vi "generate_longer_time_data.vi"(6 "new element":dbl[][](array[numeric]), 8 "Number of Samples":i32=100, 9 "横轴（显示时长）":dbl=1000.0, 10 "Sample Rate":dbl=1000.0, 11 "old array":dbl[][](array[numeric])) -> (0 "new array":dbl[][](array[numeric]), 3 "data":waveform(dbl)[](array[waveform]))   [LabVIEW 2024]
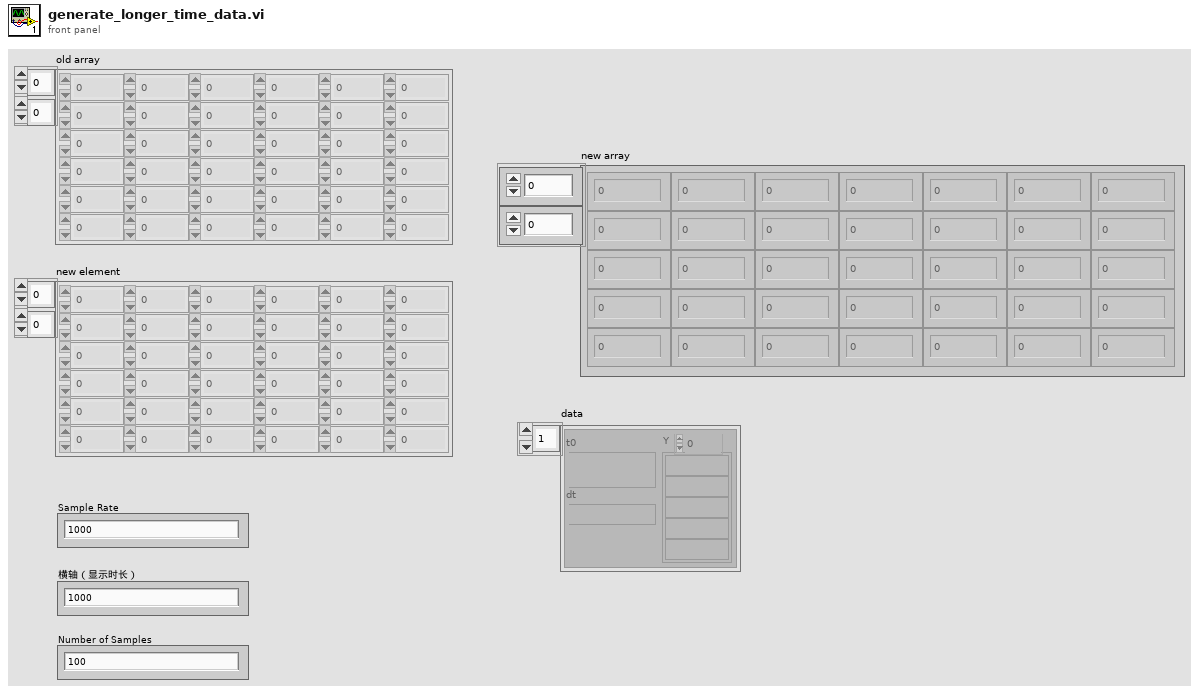
[diagram p1: front panel]
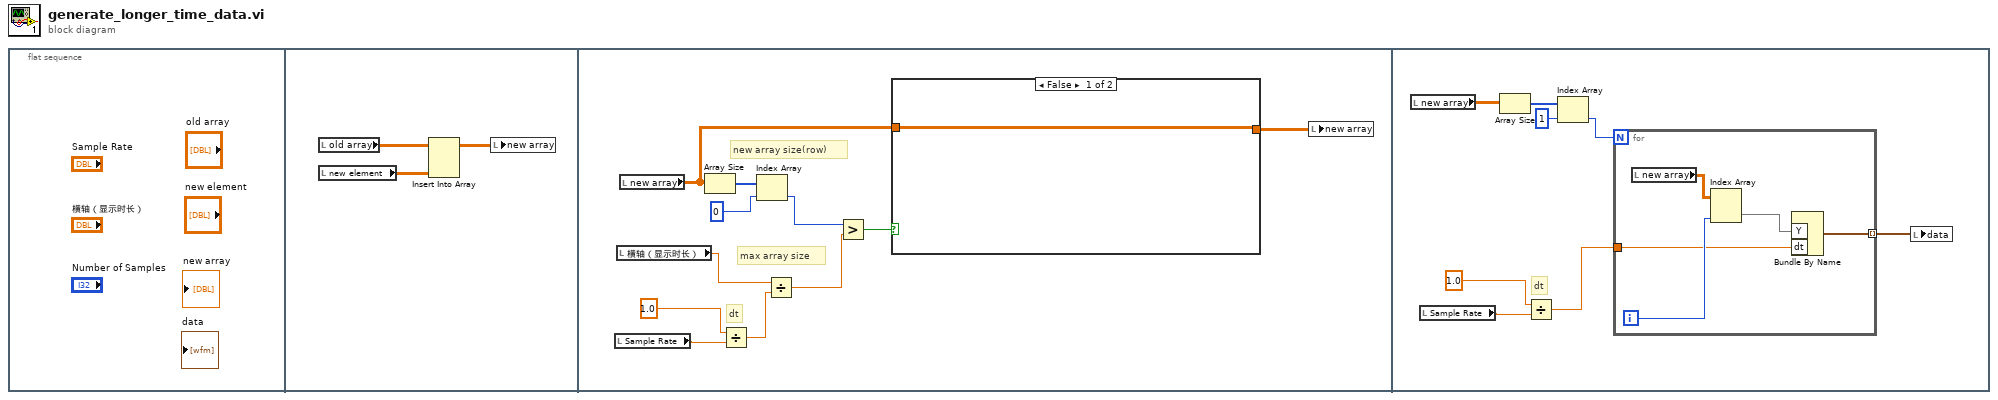
[diagram p0: block diagram]
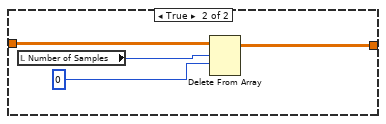
[diagram p2: hidden frame]
diagram:
  n1 = flat-sequence {
    frame #0 {
    }
    frame #1 {
      n2 = local read "old array"() -> (w1:dbl[][])
      n3 = local read "new element"() -> (w2:dbl[][])
      n4 = Insert Into Array(array=w1, new element=w2) -> (w3:dbl[][])  [unwired: 2 in]
      n5 = local write "new array"(w3) -> ()
    }
    frame #2 {
      # "new array size(row)"
      # "max array size"
      # "dt"
      n6 = local read "Sample Rate"() -> (w6:dbl)
      n7 = local read "横轴（显示时长）"() -> (w7:dbl)
      n8 = local read "new array"() -> (w13:dbl[][])
      n9 = Array Size(array=w13) -> (size(s)=w9:i32[])
      n10 = Divide(x=1.0, y=w6) -> (x/y=w8:dbl)
      n11 = Index Array(array=w9, index=0) -> (element=w10:i32)
      n12 = Divide(x=w7, y=w8) -> (x/y=w11:dbl)
      n13 = Greater?(x=w10, y=w11) -> (0:w12:bool)
      n14 = case shown="False" w12 {
        tunnel: w13 -> [w15 w19]
        tunnel: [w15 w16] -> w14
        frame False {
        }
        frame True {
          n15 = local read "Number of Samples"() -> (w18:i32)
          n16 = Delete From Array(array=w19, length=w18, index (row)=0) -> (array with subset deleted=w16:dbl[][])  [unwired: 1 in, 1 out]
        }
      }
      n17 = local write "new array"(w14) -> ()
    }
    frame #3 {
      # "dt"
      n18 = local read "new array"() -> (w27:dbl[][])
      n19 = local read "Sample Rate"() -> (w23:dbl)
      n20 = Array Size(array=w27) -> (size(s)=w26:i32[])
      n21 = Divide(x=1.0, y=w23) -> (x/y=w21:dbl)
      n22 = Index Array(array=w26, index=1) -> (element=w24:i32)
      n23 = for {
        N: w24 -> [_]
        tunnel: w21 -> [w29]
        tunnel: [w28] -> w20 mode=indexing
        i -> [w31]
        n24 = local read "new array"() -> (w32:dbl[][])
        n25 = Index Array(array=w32, index (col)=w31) -> (element=w30:dbl[])  [unwired: 1 in]
        n26 = Bundle By Name("Y"=w30, "dt"=w29) -> (w28:waveform(dbl))  [unwired: 1 in]
      }
      n27 = local write "data"(w20) -> ()
    }
  }
